vi "Dequeue Transport Element.vi"(8 "error in (no error)":errorcluster, 9 "Timeout In ms (-1)":i32=-1, 11 "QueueTransport in":refnum<class "QueueTransport.lvclass">) -> (0 "error out":errorcluster, 1 "timed out?":bool, 2 "Element":T1, 3 "QueueTransport out":refnum<class "QueueTransport.lvclass">)   [LabVIEW 2015, in "Mediator.lvlib" / "QueueTransport.lvclass"]
uses:
  QueueTransport.lvclass
  QueueTransport.lvclass/QueueTransport.ctl
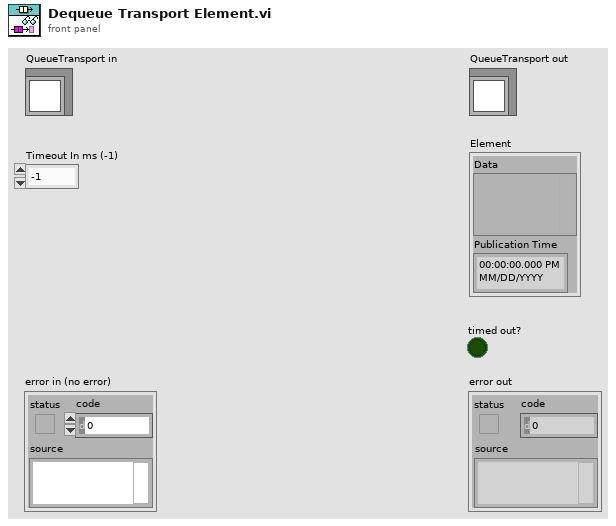
[diagram p1: front panel]
types:
  T1 = cluster{"Data":variant, "Publication Time":timestamp}
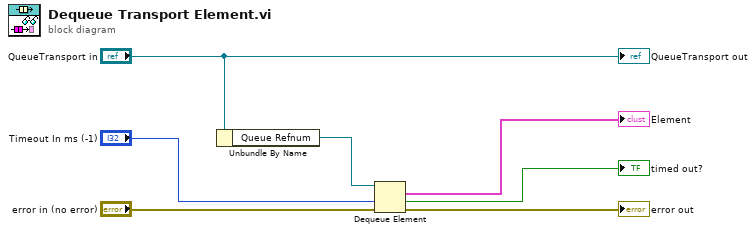
[diagram p0: block diagram]
diagram:
  n1 = Unbundle By Name("QueueTransport in") -> ("Queue Refnum"=w4:refnum<queue>)
  n2 = Dequeue Element(queue=w4, timeout in ms (-1)="Timeout In ms (-1)", error in (no error)="error in (no error)") -> (element=→"Element":T1, timed out?=→"timed out?":bool, error out=→"error out":errorcluster)  [unwired: 1 out]
  "QueueTransport out" <- "QueueTransport in"
